vi "Rolling Counter Channel.vi"(8 "error in (no error)":errorcluster, 11 "Node Ptr":T1 format="%.0x") -> (0 "error out":errorcluster)   [LabVIEW 2021, in "LIN Frame Protection Addon System Explorer.lvlib"]
uses:
  LIN Frame Protection Addon System Explorer.lvlib
  <vilib>/NI VeriStand/Custom Device API/Custom Device Item Ref.ctl
  <vilib>/NI VeriStand/Custom Device API/Custom Device API.lvlib
  Shared/LIN Frame Protection Addon Shared.lvlib
panel:
  out "Linked Path":string
  in  "Header":cluster{"Section Name":string}={"Section Name"="Custom Device Item Settings"}
  in  "Description":string
  out "Name":string
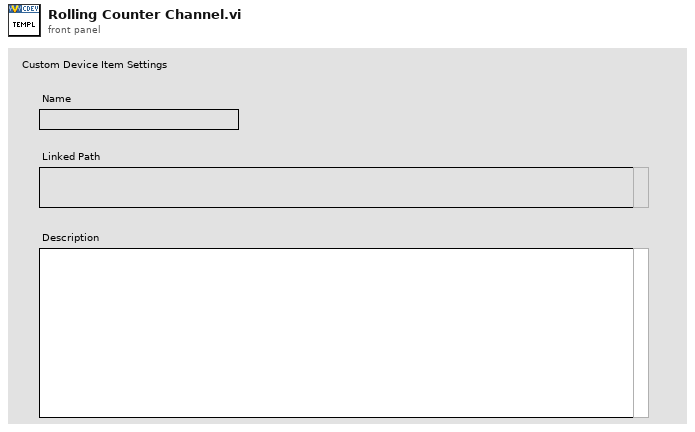
[diagram p1: front panel]
types:
  T1 = typedef "Custom Device API.lvlib/Custom Device Item Ref.ctl" = u64
  T2 = typedef "Custom Device API.lvlib/Custom Device Item Info.ctl" = cluster{"Name":string, "Is Channel":bool, "GUID":string, "Is Waveform":bool}
  T3 = typedef "LIN Frame Protection Addon Shared.lvlib/FrameConfiguration.ctl" = cluster{"Input Channels":T4[], "Schedule_SumOfDelays":dbl, "Rolling Counter Count":dbl, "PCL Count":u64, "Max Count":dbl, "Frame ID":u32, "Rolling Counter":T4, "CRC":T4, "Frame Name":string, "Cluster":string, "Database":string, "Protection Type":T5}
  T4 = typedef "LIN Frame Protection Addon Shared.lvlib/InputChannelConfiguration.ctl" = cluster{"Start Bit":i32, "Name":string, "Node Path":string, "Number of bits":i32, "Scale":dbl, "Offset":dbl, "Data Type":u32}
  T5 = typedef "LIN Frame Protection Addon Shared.lvlib/Protection Type.ctl" = enum16{"Checksum", "CRC", "None (Counter Only)"}
  T6 = typedef "Custom Device API.lvlib/Custom Device Commands.ctl" = enum16{"Default", "Item renamed", "Shutdown", "Dynamic button pressed"}
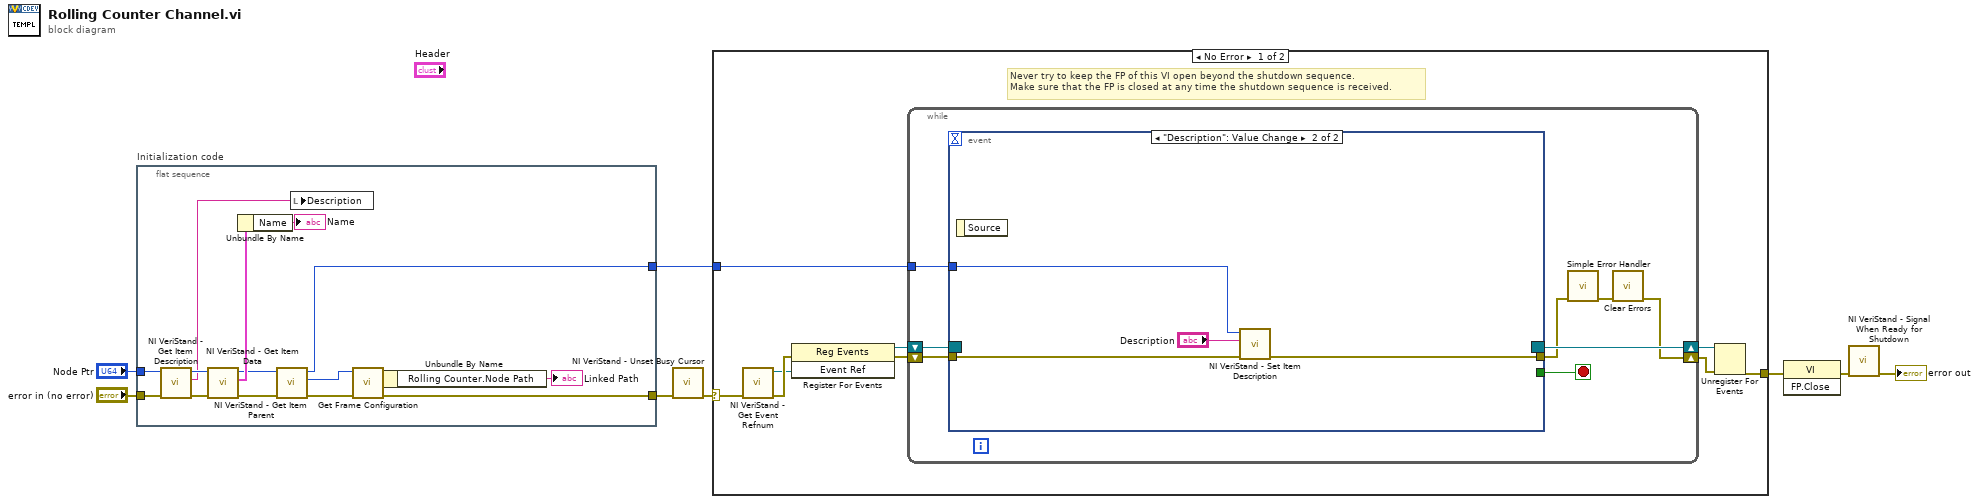
[diagram p0: block diagram]
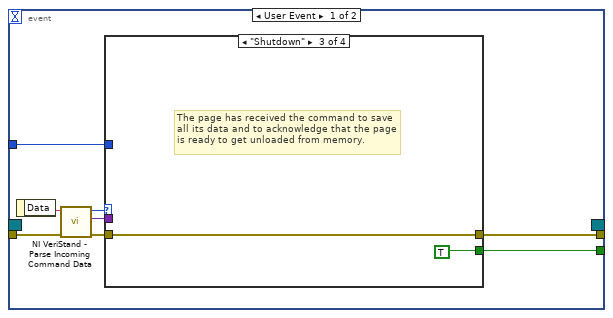
[diagram p2: hidden frame]
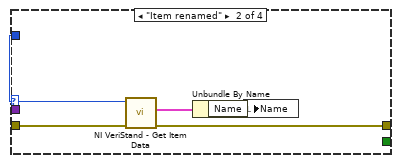
[diagram p4: hidden frame]
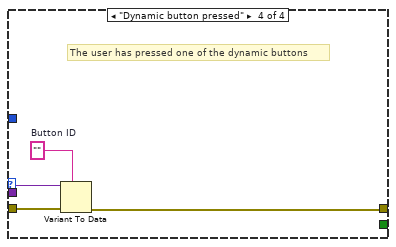
[diagram p5: hidden frame]
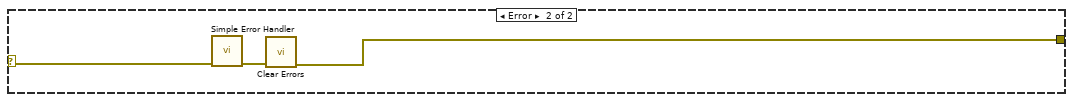
[diagram p6: hidden frame]
diagram:
  n1 = flat-sequence "Initialization code" {
    tunnel: "error in (no error)" -> [w22]
    tunnel: "Node Ptr" -> [w21]
    tunnel: [w11] -> w4
    tunnel: [w9] -> w1
    frame #0 {
      n2 = call <vilib>:"NI VeriStand - Get Item Description.vi"("error in (no error)"=w22, "Item Ref in"=w21) -> ("error out"=w19:errorcluster, "Description"=w20:string, "Item Ref out"=w23:T1)  [unwired: 7 out]
      n3 = call <vilib>:"NI VeriStand - Get Item Data.vi"("error in (no error)"=w19, "Item Ref in"=w23) -> ("error out"=w12:errorcluster, "Item Info"=w18:T2, "Item Ref out"=w10:T1)  [unwired: 7 out]
      n4 = Unbundle By Name(w18) -> ("Name"=→"Name":string)
      n5 = call <vilib>:"NI VeriStand - Get Item Parent.vi"("error in (no error)"=w12, "Item Ref in"=w10) -> ("error out"=w16:errorcluster, "Parent Ref"=w15:T1, "Item Ref out"=w9:T1)  [unwired: 6 in, 1 out]
      n6 = local write "Description"(w20) -> ()
      n7 = call "Get Frame Configuration.vi"("error in"=w16, "Parent Ref"=w15) -> ("error out"=w11:errorcluster, "Selected Channels"=w14:T3)  [unwired: 7 in, 1 out]
      n8 = Unbundle By Name(w14) -> ("Rolling Counter.Node Path"=→"Linked Path":string)
    }
  }
  n9 = call <vilib>:"NI VeriStand - Unset Busy Cursor.vi"("error in (no error)"=w4) -> ("error out"=w3:errorcluster)  [unwired: 10 out]
  n10 = case shown="No Error" w3 {
    selector: w3 -> [w24 w67]
    tunnel: [w29 w65] -> w8
    tunnel: w1 -> [w25 _]
    frame No Error {
      # "Never try to keep the FP of this VI open beyond the shutdown sequence.\nMake sure that the FP is closed at any time the shutdown sequence is received."
      n11 = call <vilib>:"NI VeriStand - Get Event Refnum.vi"("error in (no error)"=w24) -> ("error out"=w32:errorcluster, "Event Ref"=w28:refnum<user-event>)  [unwired: 9 out]
      n12 = register-events(error in=w32, w28) -> (reference out=w26:refnum<event-registration>, error out=w27:errorcluster)  [unwired: 1 in]
      n13 = while {
        tunnel: w25 -> [w36]
        shift-right: [w33] -> w30
        shift-left: w27 -> [w39]
        shift-right: [w40] -> w31
        shift-left: w26 -> [w38]
        stop <- w37 stop-if-true
        n14 = event shown="[1] \"Description\": Value Change" {
          selector: w38 -> [_ _]
          dyn-events: [_ _] -> w40
          timeout: _ -> [_ _]
          tunnel: w39 -> [w48 w63]
          tunnel: [w44 _] -> w37
          tunnel: [w43 w62] -> w35
          tunnel: w36 -> [w42 w64]
          event User Event {
            n15 = event-data() -> ("Data"=w47:string)  [unwired: 1 out]
            n16 = call <vilib>:"NI VeriStand - Parse Incoming Command Data.vi"("error in (no error)"=w48, "Incoming data"=w47) -> ("error out"=w46:errorcluster, "Outgoing data"=w41:variant, "Action"=w45:T6)  [unwired: 7 out]
            n17 = case shown="\"Shutdown\"" w45 {
              tunnel: w46 -> [w49 w54 w55 w60]
              tunnel: [_ _ TRUE _] -> w44
              tunnel: [w49 w51 w55 w57] -> w43
              tunnel: w42 -> [_ w53 _ _]
              tunnel: w41 -> [_ _ _ w59]
              frame "Default", Default {
              }
              frame "Item renamed" {
                n18 = call <vilib>:"NI VeriStand - Get Item Data.vi"("error in (no error)"=w54, "Item Ref in"=w53) -> ("error out"=w51:errorcluster, "Item Info"=w52:T2)  [unwired: 8 out]
                n19 = Unbundle By Name(w52) -> ("Name"=w50:string)
                n20 = local write "Name"(w50) -> ()
              }
              frame "Shutdown" {
                # "The page has received the command to save all its data and to acknowledge that the page is ready to get unloaded from memory."
              }
              frame "Dynamic button pressed" {
                w58 = ""  # Button ID
                # "The user has pressed one of the dynamic buttons"
                n21 = Variant To Data(error in=w60, type=w58, Variant=w59) -> (error out=w57:errorcluster)  [unwired: 1 out]
              }
            }
          }
          event "Description": Value Change {
            n22 = event-data() -> ()  [unwired: 2 out]
            n23 = call <vilib>:"NI VeriStand - Set Item Description.vi"("error in (no error)"=w63, "Description"="Description", "Item Ref in"=w64) -> ("error out"=w62:errorcluster)  [unwired: 8 out]
          }
        }
        n24 = call <vilib>:"Simple Error Handler.vi"("error in (no error)"=w35) -> ("error out"=w34:errorcluster)  [unwired: 1 in, 7 out]
        n25 = call <vilib>:"Clear Errors.vi"("error in (no error)"=w34) -> ("error out"=w33:errorcluster)  [unwired: 1 in, 5 out]
      }
      n26 = Unregister For Events(event registration refnum=w31, error in=w30) -> (error out=w29:errorcluster)
    }
    frame Error {
      n27 = call <vilib>:"Simple Error Handler.vi"("error in (no error)"=w67) -> ("error out"=w66:errorcluster)  [unwired: 1 in, 7 out]
      n28 = call <vilib>:"Clear Errors.vi"("error in (no error)"=w66) -> ("error out"=w65:errorcluster)  [unwired: 1 in, 5 out]
    }
  }
  n29 = invoke class="VI" method="FP.Close"(error in=w8) -> (error out=w7:errorcluster)  [unwired: 2 in, 2 out]
  n30 = call <vilib>:"NI VeriStand - Signal When Ready for Shutdown.vi"("error in (no error)"=w7) -> ("error out"=→"error out":errorcluster)  [unwired: 10 out]
